vi "Charger_Get Charger Record.vi"(5 "Status Refnum":T2, 6 "error in":errorcluster) -> (0 "error out":errorcluster, 1 "Charger Setpoint":dbl=7500.0 min=0.0 max=20000.0 step=100.0, 2 "address":refnum<visa-resource-name>, 3 "Charger Inputs":T1 {"setpoint" min=0.0 max=20000.0 step=100.0; "position" min=0 max=5 step=1}, 4 "position":i32 min=0 max=5 step=1)   [LabVIEW 2020]
doc: "This function gets the Charger Input values from an IPG Status reference."
uses:
  Charger_Status Refnum.ctl
  Drivers/Charger Test Set/Charger_Input Control.ctl
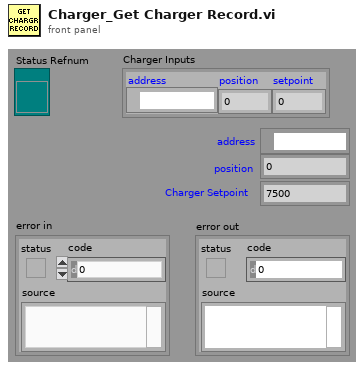
[diagram p1: front panel]
types:
  T1 = typedef "Charger_Input Control.ctl" = cluster{"address":refnum<visa-resource-name>, "position":i32, "setpoint":dbl}
  T2 = typedef "Charger_Status Refnum.ctl" = refnum<vi>
  T3 = cluster{"MICS ID":u32, "VBAT":dbl, "ChargingState":string, "VBAT Slide":dbl, "Status":string, "TemperatureLevel":dbl, "IPG_ReceivedLevel":dbl, "VBAT Target":dbl, "Charger Setpoint":dbl, "Index":i32, "Ready":bool, "Charger Inputs":T1, "MICS Inputs":cluster{"address":refnum<visa-resource-name>, "chan":u16, "ID":u32}}
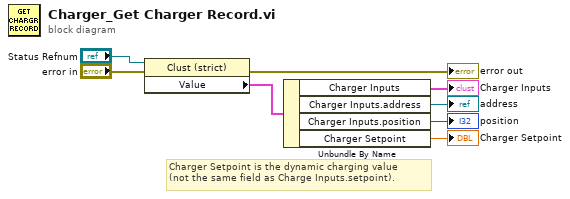
[diagram p0: block diagram]
diagram:
  # "Charger Setpoint is the dynamic charging value\n(not the same field as Charge Inputs.setpoint)."
  n1 = property class="Clust (strict)"(reference="Status Refnum", error in="error in") -> (error out=→"error out":errorcluster, "Value"=w8:T3)  [unwired: 1 out]
  n2 = Unbundle By Name(w8) -> ("Charger Inputs"=→"Charger Inputs":T1, "Charger Inputs.address"=→"address":refnum<visa-resource-name>, "Charger Inputs.position"=→"position":i32, "Charger Setpoint"=→"Charger Setpoint":dbl)
